vi "CTRE_Phoenix_Pigeon2_Open.vi"(8 "error in":errorcluster, 10 "Device Number":u8, 11 "canbus":string) -> (0 "error out":errorcluster, 3 "PigeonIMUDevRef":T1={"DeviceStatus"={"status"=FALSE, "code"=0, "source"=""}, "Device Number"=0, "Type"=352321536, "Device ID"=0, "Handle"=0, "UsageFrame"=0, "Library Path"=path ""} {"Type" items=["CAN"=352321536, "TalonSRX"=33554432]})   [LabVIEW 2020]
doc: "Opens a CTRE Pigeon2 for the given <b>Device Number</b> on the given <b>CAN Bus</b>.\n\n<b>Device Number</b> can be 0 to 63.\n<b>CAN Bus</b> is the string name of the bus. Defaults to empty string which will select the roboRIO's native CAN Bus."
uses:
  <vilib>/Rock Robotics/WPI/ThirdParty/Phoenix-LabVIEW/Pigeon IMU/CTRE_PigeonIMU_DeviceRef.ctl
  <vilib>/Rock Robotics/WPI/ThirdParty/Phoenix-LabVIEW/Pigeon IMU/CTRE_PigeonIMU_ConnectionType.ctl
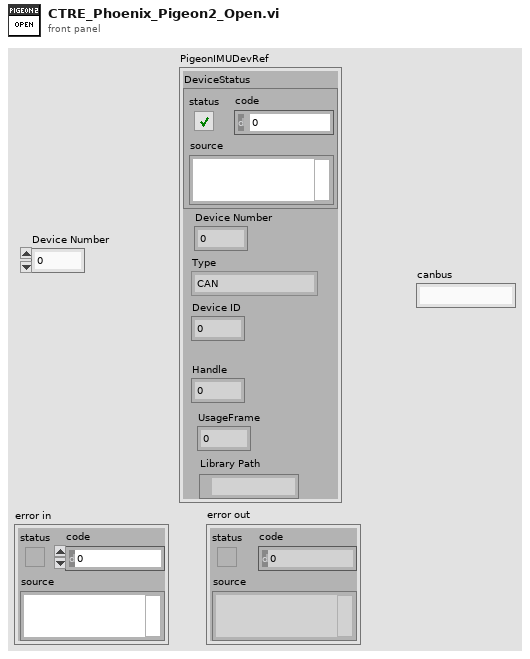
[diagram p1: front panel]
types:
  T1 = typedef "CTRE_PigeonIMU_DeviceRef.ctl" = cluster{"DeviceStatus":errorcluster, "Device Number":u8, "Type":T2, "Device ID":u32, "Handle":u64, "UsageFrame":u32, "Library Path":path}
  T2 = typedef "CTRE_PigeonIMU_ConnectionType.ctl" = u32
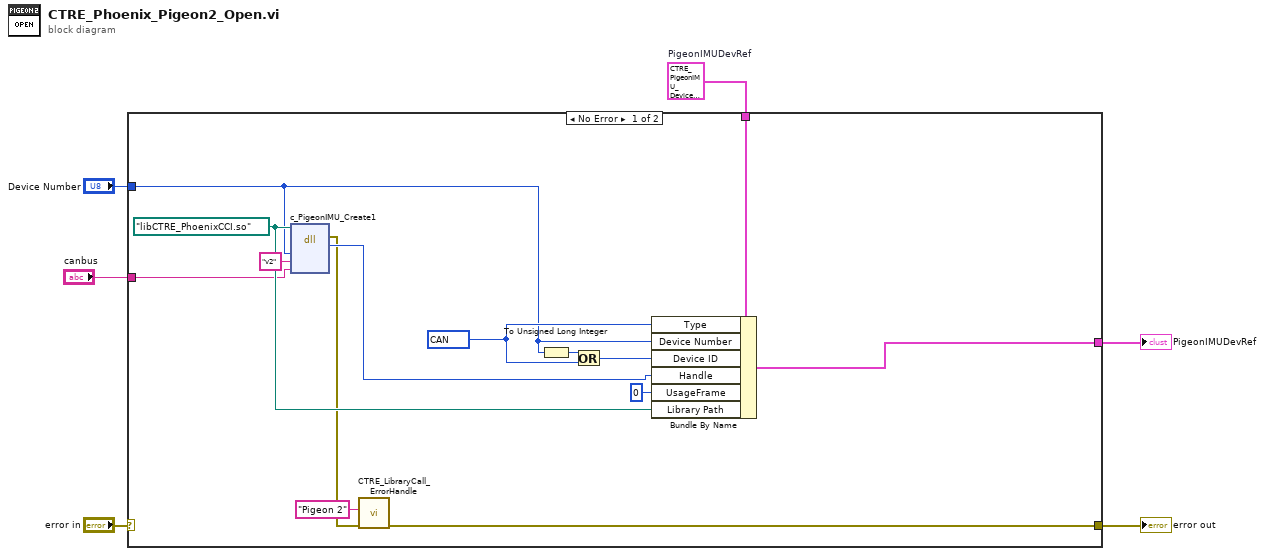
[diagram p0: block diagram]
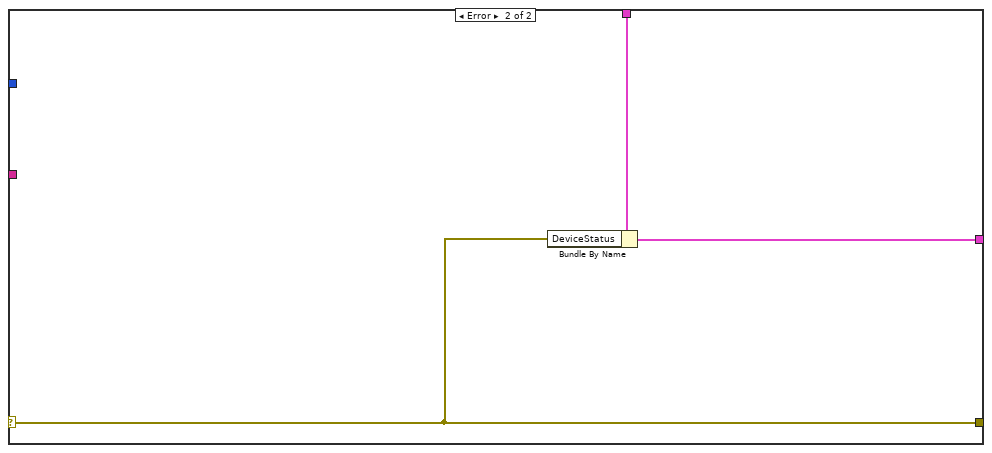
[diagram p2: hidden frame]
diagram:
  w4 = T1 {"DeviceStatus"={"status"=FALSE, "code"=0, "source"=""}, "Device Number"=0, "Type"=352321536, "Device ID"=0, "Handle"=0, "UsageFrame"=0, "Library Path"=path ""}  # PigeonIMUDevRef
  n1 = case shown="No Error" "error in" {
    selector: "error in" -> [_ w22]
    tunnel: [w13 w22] -> w5
    tunnel: w4 -> [w20 w23]
    tunnel: [w10 w21] -> w3
    tunnel: "Device Number" -> [w9 _]
    tunnel: "canbus" -> [w7 _]
    frame No Error {
      w16 = path "libCTRE_PhoenixCCI.so" ("path in")
      w17 = T2 352321536 items=["CAN"=352321536, "TalonSRX"=33554432] ("Connection Type")
      n2 = dll-call lib="?" fn="c_PigeonIMU_Create1"(path in=w16, "deviceNumber"=w9, "version"="v2", "canbus"=w7) -> (error out=w12:errorcluster, "return type"=w15:u64)  [unwired: 5 in, 1 out]
      n3 = call <vilib>:"CTRE_LibraryCall_ErrorHandle.vi"("error in"=w12, "DeviceType"="Pigeon 2") -> ("error out"=w13:errorcluster)  [unwired: 9 in]
      n4 = To Unsigned Long Integer(number=w9) -> (unsigned 32bit integer=w19:u32)
      n5 = Or(x=w19, y=w17) -> (x .or. y?=w18:T2)
      n6 = Bundle By Name(cluster=w20, "Type"=w17, "Device Number"=w9, "Device ID"=w18, "Handle"=w15, "UsageFrame"=u32 0, "Library Path"=w16) -> (w10:T1)
    }
    frame Error {
      n7 = Bundle By Name(cluster=w23, "DeviceStatus"=w22) -> (w21:T1)
    }
  }
  "error out" <- w5
  "PigeonIMUDevRef" <- w3
